vi "Set Slit Width.vi"(6 "wait for reply (T)":bool=TRUE, 8 "error in (no error)":errorcluster, 10 "Slit Width (um)":dbl, 11 "Slit":T1) -> (0 "error out":errorcluster, 1 "timed out?":bool, 2 "Reply Payload":T2)   [LabVIEW 2020, in "Spectrometer.lvlib"]
doc: "Sets the slit width of the spectrometer. If 'Wait for Reply' is true, VI executes util the slit width is set.\n_____\nCreated using Delacor QMH Event Scripter 5.0.0.112."
uses:
  Spectrometer.lvlib
  Set Slit Width (Reply Payload)--cluster.ctl
  Spectrometer-LVClass/Types/Slit.ctl
  Set Slit Width Argument--cluster.ctl
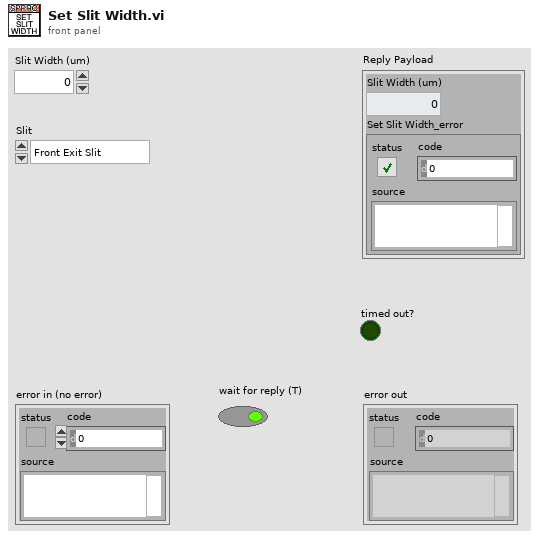
[diagram p1: front panel]
types:
  T1 = typedef "Slit.ctl" = enum16{"Front Exit Slit", "Side Exit Slit", "Front Entrance Slit", "Side Entrance Slit"}
  T2 = typedef "Spectrometer.lvlib/Set Slit Width (Reply Payload)--cluster.ctl" = cluster{"Slit Width (um)":dbl, "Set Slit Width_error":errorcluster}
  T3 = typedef "Spectrometer.lvlib/Set Slit Width Argument--cluster.ctl" = cluster{"Slit Width (um)":dbl, "Wait Notifier":refnum<notifier>, "wait for reply":bool, "Slit":T1}
  T4 = typedef "Spectrometer.lvlib/Request Events--cluster.ctl" = cluster{"Stop Module":refnum<user-event>, "Show Panel":refnum<user-event>, "Hide Panel":refnum<user-event>, "Get Module Execution Status":refnum<user-event>, "Show Diagram":refnum<user-event>, "Set Wavelength":refnum<user-event>, "Set Slit Width":refnum<user-event>, "Set Grating":refnum<user-event>, "Get Module Data":refnum<user-event>, "Set Diverter Port":refnum<user-event>}
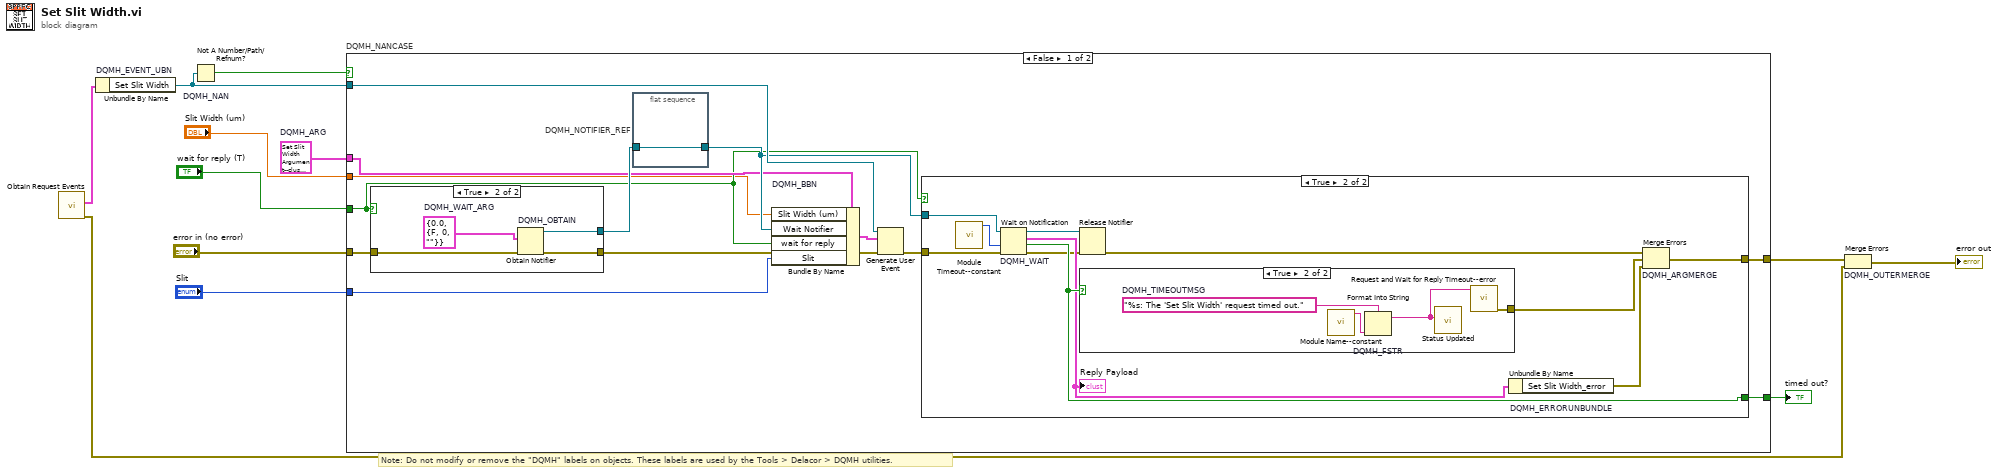
[diagram p0: block diagram]
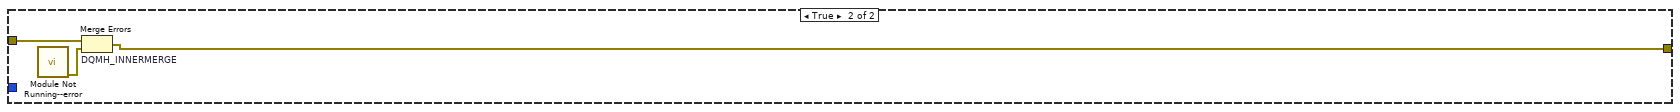
[diagram p5: hidden frame]
diagram:
  w6 = T3 {"Slit Width (um)"=0.0, "Wait Notifier"=refnum, "wait for reply"=FALSE, "Slit"=enum."Front Exit Slit"}  # DQMH_ARG
  # "Note: Do not modify or remove the \"DQMH\" labels on objects. These labels are used by the Tools > Delacor > DQMH utilities."
  n1 = call "Obtain Request Events.vi"() -> ("error out"=w3:errorcluster, "Spectrometer Request Events"=w2:T4)  [unwired: 10 in]
  n2 = Unbundle By Name "DQMH_EVENT_UBN"(w2) -> ("Set Slit Width"=w10:refnum<user-event>)
  n3 = Not A Number/Path/Refnum? "DQMH_NAN"(number/path/refnum=w10) -> (NaN/Path/Refnum?=w9:bool)
  n4 = case "DQMH_NANCASE" shown="False" w9 {
    tunnel: "error in (no error)" -> [w25 w50]
    tunnel: w10 -> [w23 _]
    tunnel: [w20 w49] -> w7
    tunnel: [w21 _] -> w8
    tunnel: w6 -> [w16 _]
    tunnel: "Slit Width (um)" -> [w14 _]
    tunnel: "wait for reply (T)" -> [w15 _]
    tunnel: "Slit" -> [w13 _]
    frame False {
      n5 = case shown="True" w15 {
        tunnel: w25 -> [w43 w47]
        tunnel: [w43 w46] -> w22
        tunnel: [_ w44] -> w18
        frame False {
        }
        frame True {
          w45 = T2 {"Slit Width (um)"=0.0, "Set Slit Width_error"={"status"=FALSE, "code"=0, "source"=""}}  # DQMH_WAIT_ARG
          n6 = Obtain Notifier "DQMH_OBTAIN"(notification data type=w45, error in (no error)=w47) -> (notifier out=w44:refnum<notifier>, error out=w46:errorcluster)  [unwired: 2 in, 1 out]
        }
      }
      n7 = flat-sequence "DQMH_NOTIFIER_REF" {
        tunnel: w18 -> [w26]
        tunnel: [w26] -> w17
        frame #0 {
        }
      }
      n8 = Bundle By Name "DQMH_BBN"(cluster=w16, "Slit Width (um)"=w14, "Wait Notifier"=w17, "wait for reply"=w15, "Slit"=w13) -> (w19:T3)
      n9 = Generate User Event(user event=w23, event data cluster=w19, error in=w22) -> (error out=w24:errorcluster)  [unwired: 1 in, 1 out]
      n10 = case shown="True" w15 {
        tunnel: w24 -> [w27 w38]
        tunnel: w17 -> [_ w37]
        tunnel: [_ w35] -> w21
        tunnel: [w27 w34] -> w20
        frame False {
        }
        frame True {
          n11 = call "Module Timeout--constant.vi"() -> ("Module Timeout"=w28:i32)  [unwired: 11 in]
          n12 = Wait on Notification "DQMH_WAIT"(notifier=w37, timeout in ms (-1)=w28, error in (no error)=w38) -> (notifier out=w36:refnum<notifier>, notification=w33:T2, timed out?=w35:bool, error out=w32:errorcluster)  [unwired: 1 in]
          "Reply Payload" <- w33
          n13 = Release Notifier(notifier=w36, error in (no error)=w32) -> (error out=w31:errorcluster)  [unwired: 1 in, 2 out]
          n14 = case shown="True" w35 {
            tunnel: [_ w40] -> w29
            frame False {
            }
            frame True {
              w42 = "%s: The 'Set Slit Width' request timed out."  # DQMH_TIMEOUTMSG
              n15 = call "Module Name--constant.vi"() -> ("Module Name"=w39:string)  [unwired: 11 in]
              n16 = Format Into String "DQMH_FSTR"(format string=w42, w39) -> (resulting string=w41:string)  [unwired: 2 in, 1 out]
              n17 = call "Status Updated.vi"("Status"=w41) -> ()  [unwired: 10 in, 1 out]
              n18 = call "Request and Wait for Reply Timeout--error.vi"("Error Message"=w41) -> ("error out"=w40:errorcluster)  [unwired: 10 in]
            }
          }
          n19 = Unbundle By Name "DQMH_ERRORUNBUNDLE"(w33) -> ("Set Slit Width_error"=w30:errorcluster)
          n20 = Merge Errors "DQMH_ARGMERGE"(w31, w29, w30) -> (w34:errorcluster)
        }
      }
    }
    frame True {
      n21 = call "Module Not Running--error.vi"() -> ("error out"=w48:errorcluster)  [unwired: 11 in]
      n22 = Merge Errors "DQMH_INNERMERGE"(w50, w48) -> (w49:errorcluster)
    }
  }
  "timed out?" <- w8
  n23 = Merge Errors "DQMH_OUTERMERGE"(w7, w3) -> (→"error out":errorcluster)
